vi "Inv_Mpemba1_QPDcali.vi"() -> ()   [LabVIEW 2019]
uses:
  <vilib>/eio/EIONode/EIONode.xnode
  <vilib>/rvi/eio/common/nirviEmuTemplateMethod_errors.vi
  <vilib>/eio/EIOPropertyNode/EIOPropertyNode.xnode
  <vilib>/rvi/eio/common/nirviEmuTemplatePropertyGet_errors.vi
  <vilib>/rvi/eio/common/nirviEmuTemplatePropertyGet_noerrors.vi
  <vilib>/rvi/eio/common/nirviEmuTemplatePropertySet_errors.vi
  <vilib>/rvi/eio/common/nirviEmuTemplatePropertySet_noerrors.vi
  <vilib>/rvi/DataTransferAndStorage/Container/XNode/niFpgaContainer.xnode
  <vilib>/rvi/FIFO/Fifo_Resource/nirvififoEmulationWrite.vi
  <vilib>/rvi/FIFO/Fifo_Resource/nirvififoEmulationRead.vi
  <vilib>/rvi/interface/RandomDataEmulation/nirviRandomDataFpgaReadWriteTemplate.vi
panel:
  in  "V_offset":sgl
  in  "Calibration":T1
  in  "Bias":sgl
  out "num of cycles":sgl
  in  "Xmin":sgl=-1.0
  in  "Fmax":sgl
  out "Fx out/Xcorr":sgl
  in  "Xmax":sgl=50.0
  out "Xpot":sgl format="%.2f"
  in  "Temp":i8(ring) items=["Cold", "Warm", "Hot"]
  in  "cdfnorm":sgl
  out "Saveloop":u32
  in  "Enum":enum8{"No FB", "FB"}(ring)
  in  "MobX(px/V)":sgl
  in  "1/Xcali":sgl
  in  "Feedback parameters":T2
  in  "DX":sgl
  in  "DW":cluster{"xm":sgl, "Eb":sgl, "Tau":sgl, "dE":sgl}={"xm"=0.0, "Eb"=0.0, "Tau"=50.0, "dE"=0.0}
  in  "Xmean":sgl
  in  "Calibration ON/OFF":bool
  in  "Frequency":u32=100000
  in  "wait time":sgl=35.0
  in  "Triangle wave":T3={"signal offset_X"=5.0, "Scale X"=0.0, "signal offset_Y"=5.0, "Scale Y"=0.0, "Phase Shift"=30}
  in  "Xoffset":sgl
  in  "Yoffset":sgl
  in  "sum_offset":sgl
  in  "Normalize signal":bool=TRUE
  in  "FB Time":u8=5 caption="Feedback loop time"
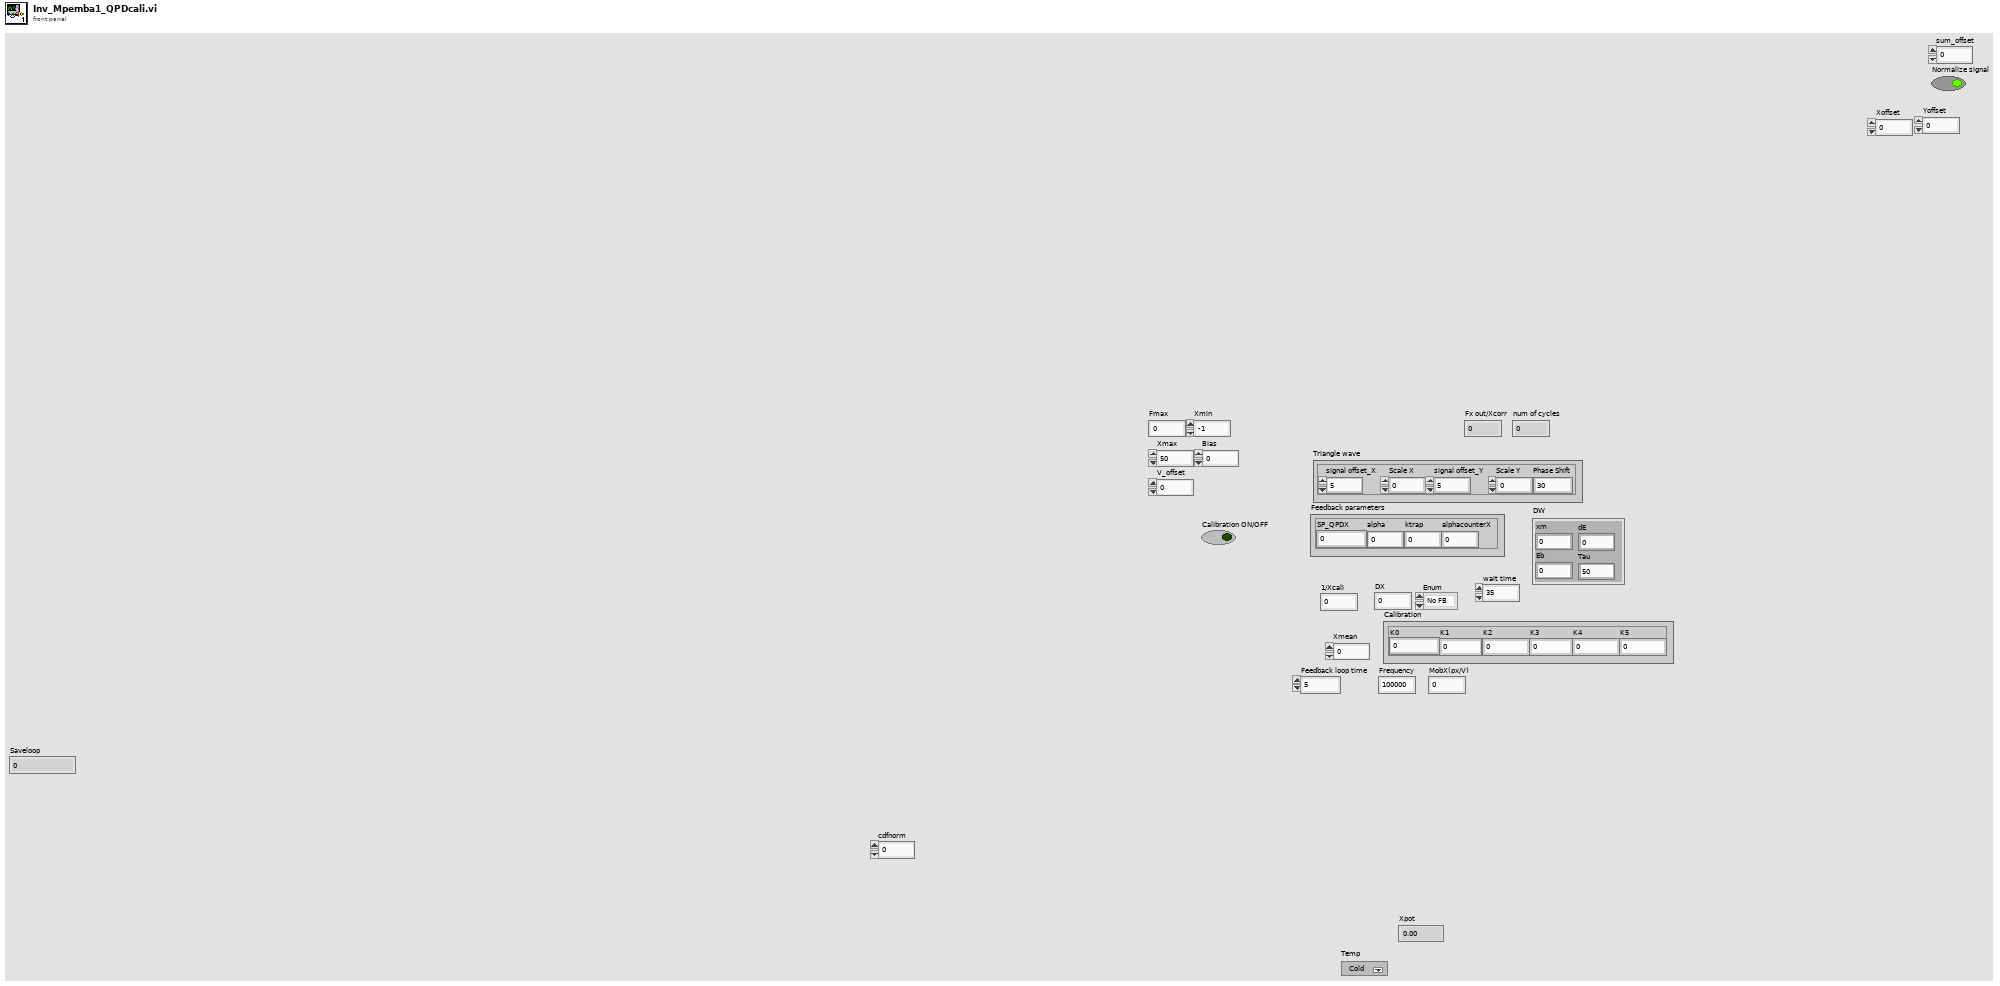
[diagram p1: front panel]
types:
  T1 = cluster{"K0":sgl, "K1":sgl, "K2":sgl, "K3":sgl, "K4":sgl, "K5":sgl}
  T2 = cluster{"SP_QPDX":sgl, "alpha":sgl, "ktrap":sgl, "alphacounterX":sgl}
  T3 = cluster{"signal offset_X":sgl, "Scale X":sgl, "signal offset_Y":sgl, "Scale Y":sgl, "Phase Shift":u32}
  T4 = enum8{"+/- 10 V", "+/- 5 V", "+/- 2 V", "+/- 1 V"}
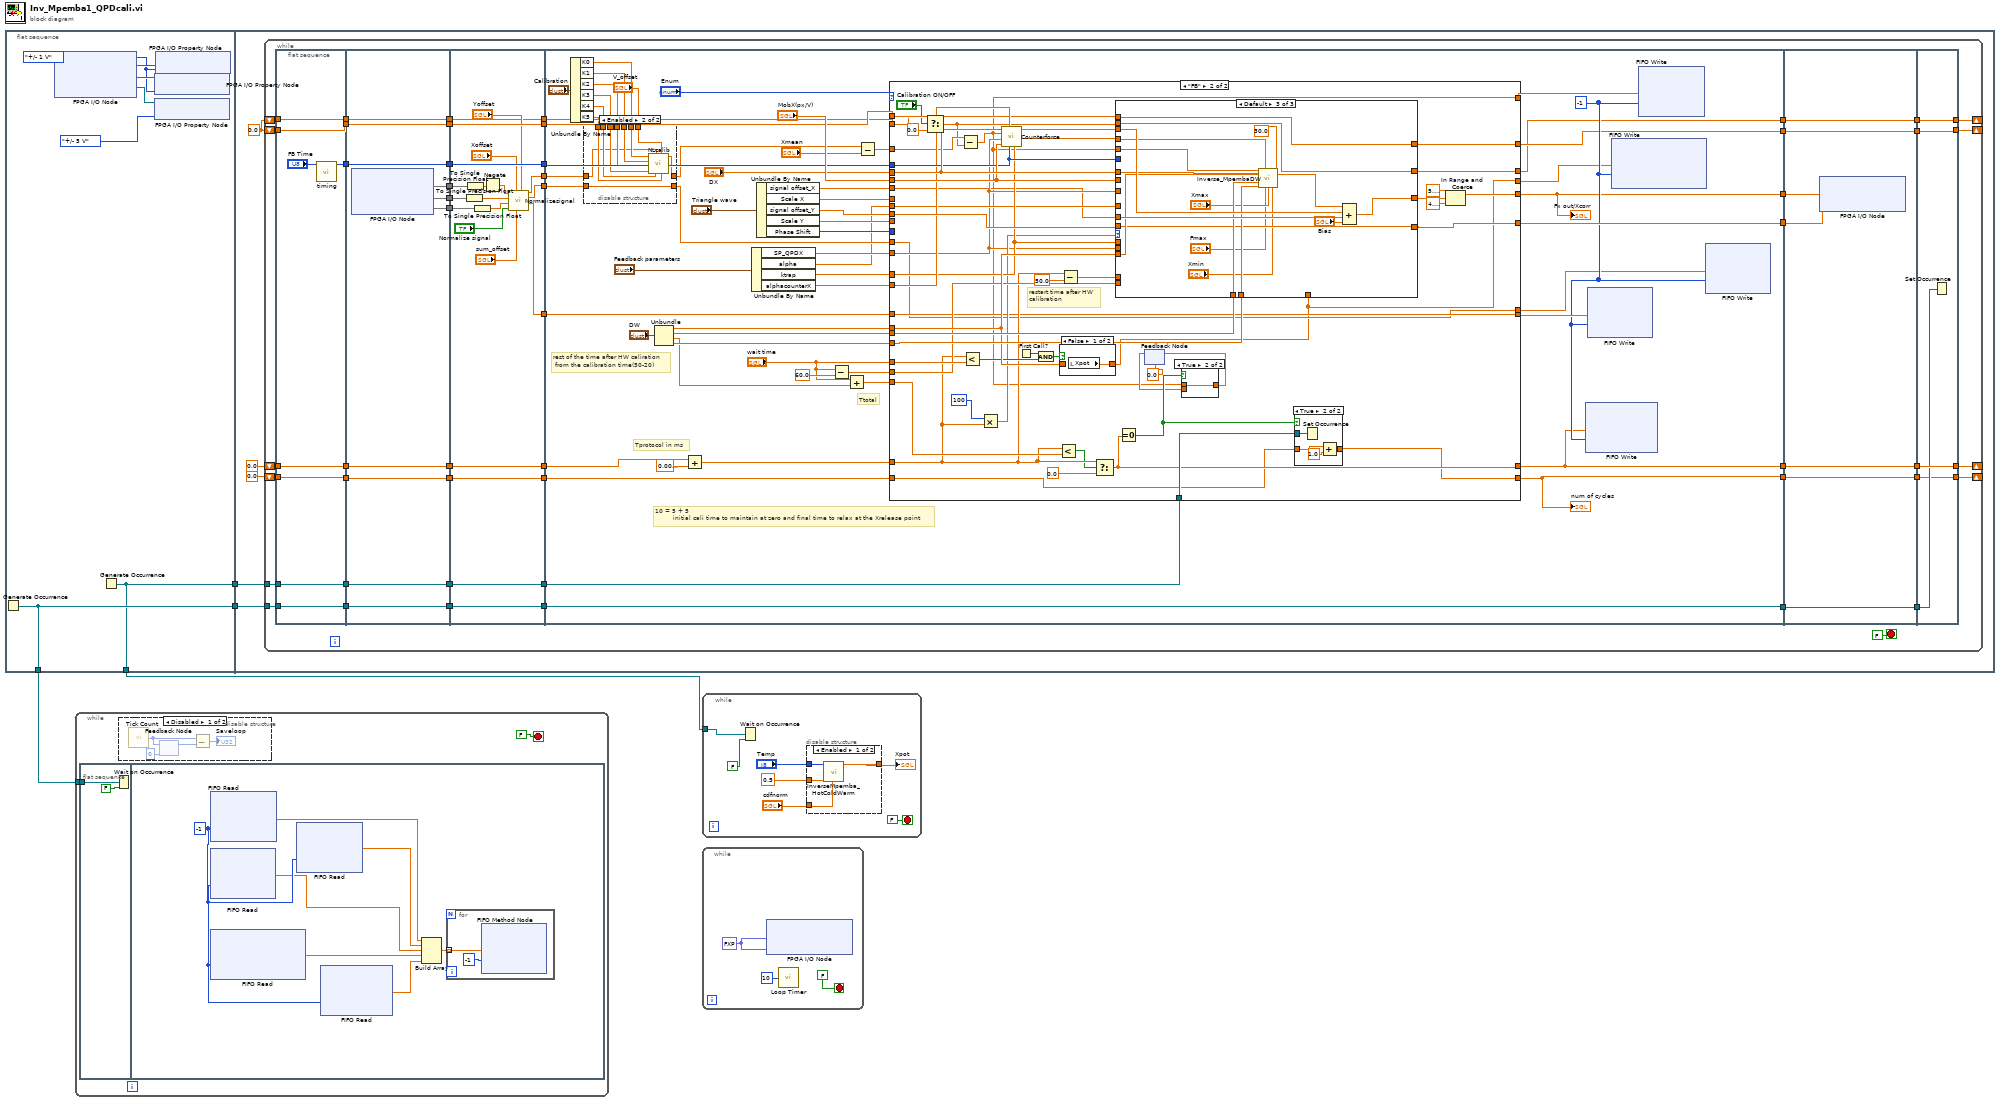
[diagram p0: block diagram]
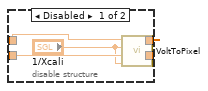
[diagram p2: hidden frame]
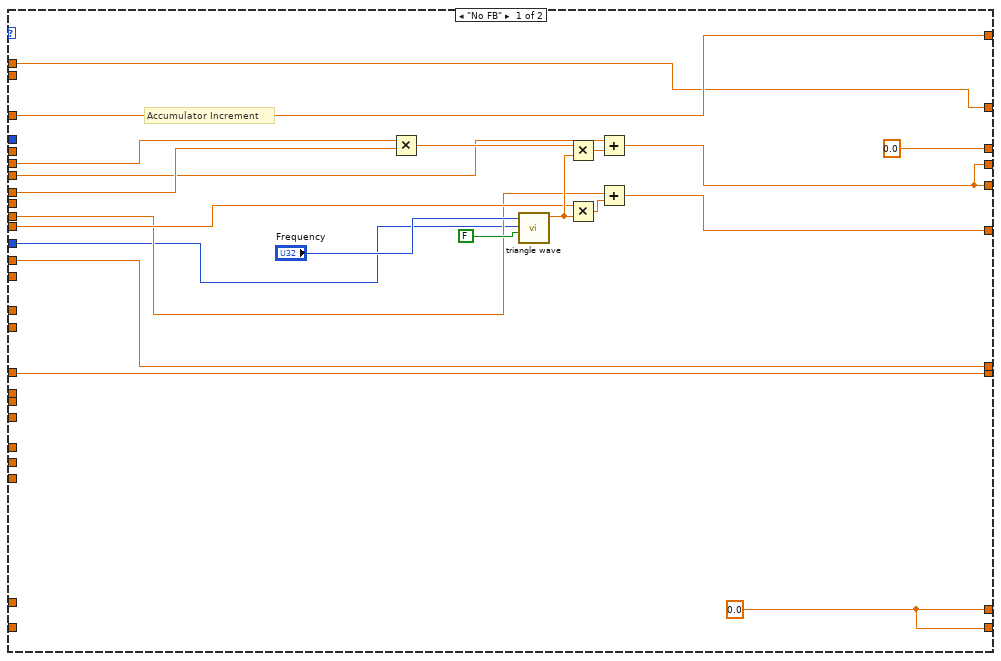
[diagram p3: hidden frame]
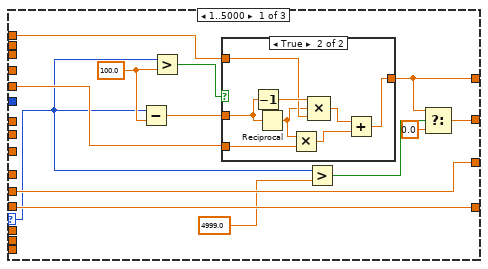
[diagram p4: hidden frame]
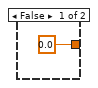
[diagram p5: hidden frame]
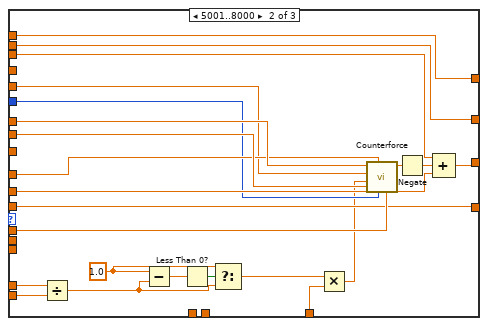
[diagram p6: hidden frame]
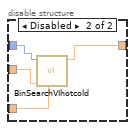
[diagram p11: hidden frame]
diagram:
  n1 = flat-sequence {
    tunnel: [w6] -> w2
    tunnel: [w5] -> w1
    tunnel: [w6] -> w4
    tunnel: [w5] -> w3
    tunnel: w2 -> [w16]
    tunnel: w1 -> [w15]
    frame #0 {
      w8 = T4."+/- 1 V" ("Voltage Range")
      n2 = Generate Occurrence() -> (w6:refnum<k4>)
      n3 = xnode "FPGA I/O Node"() -> ("FPGA I/O Out"=w11:refnum<k21>, "FPGA I/O Out"=w9:refnum<k21>, "FPGA I/O Out"=w10:refnum<k21>)  [unwired: 3 in, 3 out]
      n4 = Generate Occurrence() -> (w5:refnum<k4>)
      n5 = xnode "FPGA I/O Property Node"("FPGA I/O In"=w9, "Voltage Range"=w8) -> ()  [unwired: 1 out]
      n6 = xnode "FPGA I/O Property Node"("FPGA I/O In"=w10, "Voltage Range"=T4."+/- 5 V") -> ()  [unwired: 1 out]
      n7 = xnode "FPGA I/O Property Node"("FPGA I/O In"=w11, "Voltage Range"=w8) -> ()  [unwired: 1 out]
    }
    frame #1 {
      w12 = sgl 0.0
      n8 = while {
        tunnel: w16 -> [w47]
        shift-right: [w52] -> _
        shift-left: sgl 0.0 -> [w51]
        tunnel: w15 -> [w38]
        shift-right: [w35] -> _
        shift-left: w12 -> [w33]
        shift-right: [w28] -> _
        shift-left: sgl 0.0 ("f") -> [w26]
        shift-right: [w21] -> _
        shift-left: w12 -> [w20]
        stop <- FALSE ("stop") stop-if-true
        n9 = flat-sequence {
          tunnel: [w73] -> w55
          tunnel: w51 -> [w72]
          tunnel: [w72] -> w50
          tunnel: w47 -> [w71]
          tunnel: [w71] -> w46
          tunnel: [w70] -> w39
          tunnel: w38 -> [w70]
          tunnel: [w69] -> w34
          tunnel: w33 -> [w69]
          tunnel: [w68] -> w27
          tunnel: w26 -> [w68]
          tunnel: w20 -> [w67]
          tunnel: [w67] -> w19
          tunnel: [w84] -> w65
          tunnel: [w83] -> w63
          tunnel: [w82] -> w61
          tunnel: [w81] -> w56
          tunnel: w55 -> [w81]
          tunnel: w50 -> [w80]
          tunnel: [w80] -> w49
          tunnel: w46 -> [w79]
          tunnel: [w79] -> w45
          tunnel: [w78] -> w40
          tunnel: w39 -> [w78]
          tunnel: w34 -> [w77]
          tunnel: [w77] -> w31
          tunnel: w27 -> [w76]
          tunnel: [w76] -> w25
          tunnel: w19 -> [w75]
          tunnel: [w75] -> w18
          tunnel: w65 -> [w92]
          tunnel: [w104] -> w64
          tunnel: w63 -> [w91]
          tunnel: [w103] -> w62
          tunnel: w61 -> [w89]
          tunnel: [w102] -> w60
          tunnel: [w105] -> w57
          tunnel: w56 -> [w105]
          tunnel: w49 -> [w101]
          tunnel: [w101] -> w48
          tunnel: w45 -> [w100]
          tunnel: [w100] -> w44
          tunnel: [w99] -> w41
          tunnel: w40 -> [w99]
          tunnel: [w97] -> w32
          tunnel: w31 -> [w97]
          tunnel: w25 -> [w96]
          tunnel: [w96] -> w24
          tunnel: w18 -> [w87]
          tunnel: [w87] -> w17
          tunnel: w64 -> [w159]
          tunnel: w62 -> [w158]
          tunnel: w60 -> [w153]
          tunnel: [w114] -> w59
          tunnel: [w163] -> w58
          tunnel: w57 -> [w160]
          tunnel: [w133] -> w54
          tunnel: w48 -> [w155]
          tunnel: w44 -> [w146]
          tunnel: [w146] -> w42
          tunnel: w41 -> [w140]
          tunnel: [w135] -> w37
          tunnel: w32 -> [w134]
          tunnel: [w116] -> w30
          tunnel: w24 -> [w132]
          tunnel: [w118] -> w23
          tunnel: w17 -> [w117]
          tunnel: w58 -> [w328]
          tunnel: w59 -> [w329]
          tunnel: w54 -> [w327]
          tunnel: [w327] -> w53
          tunnel: [w326] -> w43
          tunnel: w42 -> [w326]
          tunnel: w37 -> [w325]
          tunnel: [w325] -> w36
          tunnel: w30 -> [w324]
          tunnel: [w324] -> w29
          tunnel: w23 -> [w323]
          tunnel: [w323] -> w22
          tunnel: w53 -> [w334]
          tunnel: [w334] -> w52
          tunnel: w43 -> [w333]
          tunnel: [w332] -> w35
          tunnel: w36 -> [w332]
          tunnel: w29 -> [w331]
          tunnel: [w331] -> w28
          tunnel: w22 -> [w330]
          tunnel: [w330] -> w21
          frame #0 {
            n10 = call "timing.vi"("Feedback loop time"="FB Time") -> ("Feedback Loop time"=w73:u32)  [unwired: 10 in]
          }
          frame #1 {
            n11 = xnode "FPGA I/O Node"() -> ("Connector1/AI2"=w84, "Connector1/AI4"=w83, "Connector1/AI5"=w82)  [unwired: 3 in, 3 out]
          }
          frame #2 {
            n12 = To Single Precision Float(number=w91) -> (single precision float=w90:sgl)
            n13 = To Single Precision Float(number=w92) -> (single precision float=w86:sgl)
            n14 = To Single Precision Float(number=w89) -> (single precision float=w88:sgl)
            n15 = Negate(x=w86) -> (-x=w85:sgl)
            n16 = call "Normalizesignal.vi"("Yoffset"="Yoffset", "sum_offset"="sum_offset", "Xoffset"="Xoffset", "Normalize signal"="Normalize signal", "Sum"=w88, "Y"=w90, "X"=w85) -> ("Sum"=w102:sgl, "Y"=w103:sgl, "X"=w104:sgl)  [unwired: 2 in]
          }
          frame #3 {
            w136 = -1 ("Timeout")
            # "rest of the time after HW caliration\n from the calibration time(50-20)"
            # "10 = 5 + 5\n         initial cali time to maintain at zero and final time to relax at the Xrelease point"
            # "Tprotocol in ms"
            # "Ttotal"
            n17 = Unbundle By Name("Calibration") -> ("K0"=w111:sgl, "K1"=w110:sgl, "K2"=w109:sgl, "K3"=w108:sgl, "K4"=w107:sgl, "K5"=w106:sgl)
            n18 = disable-structure shown="Enabled" {
              disable-tunnel: w159 -> [w168 w170]
              disable-tunnel: w158 -> [w167 w178]
              disable-tunnel: [w166 w178] -> w157
              disable-tunnel: [w165 w169] -> w143
              disable-tunnel: "V_offset" -> [_ w177]
              disable-tunnel: w111 -> [_ w176]
              disable-tunnel: w110 -> [_ w175]
              disable-tunnel: w109 -> [_ w174]
              disable-tunnel: w108 -> [_ w173]
              disable-tunnel: w107 -> [_ w172]
              disable-tunnel: w106 -> [_ w171]
              frame Disabled {
                n19 = call "VoltToPixel.vi"("1/(QPDY/px)"="1/Xcali", "Normalized Y"=w167, "1/(QPDX/px)"="1/Xcali", "Normalized X"=w168) -> ("Ypx"=w166:sgl, "Xpx"=w165:sgl)  [unwired: 6 in]
              }
              frame Enabled {
                n20 = call "NLcalib.vi"("K5"=w171, "V_offset"=w177, "K4"=w172, "Volt QPD"=w170, "K3"=w173, "K2"=w174, "K1"=w175, "K0"=w176) -> ("pixels"=w169:sgl)  [unwired: 3 in]
              }
            }
            n21 = Unbundle("DW") -> ("xm"=w141:sgl, "Eb"=w154:sgl, "Tau"=w120:sgl, "dE"=w148:sgl)
            n22 = Add(x=w155, y=sgl 0.01) -> (x+y=w147:sgl)
            n23 = Unbundle By Name("Feedback parameters") -> ("SP_QPDX"=w124:sgl, "alpha"=w121:sgl, "ktrap"=w122:sgl, "alphacounterX"=w123:sgl)
            n24 = Unbundle By Name("Triangle wave") -> ("signal offset_X"=w128:sgl, "Scale X"=w130:sgl, "signal offset_Y"=w127:sgl, "Scale Y"=w129:sgl, "Phase Shift"=w126:u32)
            n25 = Subtract(x="wait time", y=sgl 60.0) -> (x-y=w139:sgl)
            n26 = Add(x="wait time", y=w120) -> (x+y=w156:sgl)
            n27 = Subtract(x=w143, y="Xmean") -> (x-y=w151:sgl)
            n28 = case shown="\"FB\"" "Enum" {
              tunnel: w151 -> [w196 w204]
              tunnel: [w179 w224] -> w114
              tunnel: [w190 w216] -> w163
              tunnel: [w196 w202] -> w150
              tunnel: [w198 w209] -> w149
              tunnel: w153 -> [w198 w209]
              tunnel: w157 -> [w197 w206]
              tunnel: [w197 w206] -> w119
              tunnel: "MobX(px/V)" -> [w189 w247]
              tunnel: w160 -> [_ w230]
              tunnel: "DX" -> [_ w248]
              tunnel: w141 -> [_ w243]
              tunnel: w154 -> [_ w249]
              tunnel: w147 -> [_ w218]
              tunnel: w156 -> [_ w232]
              tunnel: [w181 w241] -> w133
              tunnel: w148 -> [_ w246]
              tunnel: w140 -> [_ w242]
              tunnel: "wait time" -> [_ w238]
              tunnel: w139 -> [_ w229]
              tunnel: [w188 w200] -> w135
              tunnel: w134 -> [w188 w212]
              tunnel: [w181 w226] -> w116
              tunnel: w132 -> [_ w225]
              tunnel: w130 -> [w186 _]
              tunnel: w129 -> [w185 _]
              tunnel: w128 -> [w184 w205]
              tunnel: w127 -> [w183 w223]
              tunnel: w126 -> [w182 _]
              tunnel: w124 -> [_ w213]
              tunnel: w123 -> [_ w222]
              tunnel: w122 -> [_ w221]
              tunnel: w121 -> [_ w220]
              tunnel: [sgl 0.0 ("f") w201] -> w118
              tunnel: w117 -> [_ w207]
              tunnel: [w179 w199] -> w115
              frame "No FB" {
                w181 = sgl 0.0 ("f")
                # "Accumulator Increment"
                n29 = Multiply(x=w189, y=w186) -> (x*y=w194:sgl)
                n30 = call "triangle wave.vi"("Reset Accumulator_TW"=FALSE, "phase shift"=w182, "Frequency"="Frequency") -> ("Tri wave out"=w191:sgl)  [unwired: 8 in]
                n31 = Multiply(x=w194, y=w191) -> (x*y=w193:sgl)
                n32 = Multiply(x=w185, y=w191) -> (x*y=w195:sgl)
                n33 = Add(x=w184, y=w193) -> (x+y=w179:sgl)
                n34 = Add(x=w183, y=w195) -> (x+y=w190:sgl)
              }
              frame "FB" {
                # "restart time after HW\ncalibration"
                n35 = Select(t=w207, s="Calibration ON/OFF", f=sgl 0.0) -> (s? t:f=w203:sgl)
                n36 = Subtract(x=w204, y=w203) -> (x-y=w202:sgl)
                n37 = Less?(x=w218, y=w238) -> (x < y?=w234:bool)
                n38 = Multiply(x=i16 100, y=w218) -> (x*y=w217:sgl)
                n39 = call "Counterforce.vi"("ktrap"=w221, "Ts"=w230, "alphacounterX"=w222, "mobX(px/V)"=w247, "SP_X"=w213, "Xpx"=w202, "Dx"=w248) -> ("ktrap*mob"=w239:sgl, "counter Force"=w240:sgl)  [unwired: 2 in, 1 out]
                n40 = First Call?() -> (First Call?: T/F=w245:bool)
                n41 = And(x=w245, y=w234) -> (x .and. y?=w244:bool)
                n42 = Less?(x=w218, y=w232) -> (x < y?=w208:bool)
                n43 = case shown="False" w244 {
                  tunnel: [w321 w322] -> w199
                  tunnel: w243 -> [_ w322]
                  frame False {
                    n44 = local read "Xpot"() -> (w321:sgl)
                  }
                  frame True {
                  }
                }
                n45 = Subtract(x=w218, y=sgl 50.0) -> (x-y=w227:sgl)
                n46 = Select(t=w218, s=w208, f=sgl 0.0) -> (s? t:f=w241:sgl)
                n47 = case shown="Default" w217 {
                  selector: w217 -> [w256 _ _]
                  tunnel: w202 -> [w258 w275 w305]
                  tunnel: w248 -> [_ w295 w300]
                  tunnel: w247 -> [_ w294 _]
                  tunnel: [w257 w293 w308] -> w219
                  tunnel: [w262 w289 w307] -> w216
                  tunnel: w221 -> [_ w290 _]
                  tunnel: w223 -> [w262 w289 w307]
                  tunnel: w205 -> [w257 w286 w313]
                  tunnel: w220 -> [_ w288 _]
                  tunnel: w243 -> [_ _ w311]
                  tunnel: w249 -> [_ _ w310]
                  tunnel: w240 -> [_ w287 w312]
                  tunnel: w239 -> [_ _ w302]
                  tunnel: w246 -> [_ _ w309]
                  tunnel: w213 -> [_ _ _]
                  tunnel: [w253 w276 w306] -> w200
                  tunnel: w212 -> [w259 w276 w306]
                  tunnel: w230 -> [_ w285 _]
                  tunnel: w199 -> [_ w284 _]
                  tunnel: w227 -> [_ w278 _]
                  tunnel: w229 -> [_ w277 _]
                  tunnel: w213 -> [_ _ _]
                  tunnel: [w251 w274 w303] -> w201
                  tunnel: w203 -> [_ w274 w303]
                  frame 1..5000 {
                    w263 = sgl 100.0 ("y")
                    n48 = Subtract(x=w256, y=w263) -> (x-y=w260:sgl)
                    n49 = Greater?(x=w256, y=w263) -> (0:w261:bool)
                    n50 = case shown="True" w261 {
                      tunnel: [sgl 0.0 w266] -> w253
                      tunnel: w260 -> [_ w272]
                      tunnel: w259 -> [_ w270]
                      tunnel: w258 -> [_ w269]
                      frame False {
                      }
                      frame True {
                        n51 = Decrement(x=w272) -> (x-1=w271:sgl)
                        n52 = Reciprocal(x=w272) -> (1/x=w265:sgl)
                        n53 = Multiply(x=w265, y=w269) -> (x*y=w267:sgl)
                        n54 = Compound Arithmetic op=MULTIPLY(w271, w265, w270) -> (w268:sgl)
                        n55 = Add(x=w268, y=w267) -> (x+y=w266:sgl)
                      }
                    }
                    n56 = Greater?(x=w256, y=sgl 4999.0) -> (0:w254:bool)
                    n57 = Select(t=w253, s=w254, f=sgl 0.0) -> (s? t:f=w251:sgl)
                  }
                  frame 5001..8000 {
                    w280 = sgl 1.0 ("y")
                    n58 = Divide(x=w278, y=w277) -> (x/y=w279:sgl)
                    n59 = Subtract(x=w280, y=w279) -> (x-y=w281:sgl)
                    n60 = Less Than 0?(x=w281) -> (x < 0?=w282:bool)
                    n61 = Select(t=w280, s=w282, f=w279) -> (s? t:f=w283:sgl)
                    n62 = Multiply(x=w283, y=w284) -> (x*y=w273:sgl)
                    n63 = call "Counterforce.vi"("ktrap"=w290, "Ts"=w285, "alphacounterX"=w288, "mobX(px/V)"=w294, "SP_X"=w273, "Xpx"=w275, "Dx"=w295) -> ("counter Force"=w292:sgl)  [unwired: 2 in, 2 out]
                    n64 = Negate(x=w292) -> (-x=w291:sgl)
                    n65 = Compound Arithmetic op=ADD(w287, w291, w286) -> (w293:sgl)
                  }
                  frame Default {
                    n66 = call "Inverse_MpembaDW.vi"("Xpos"=w305, "ktrap*mob"=w302, 2:w300, 4:sgl 30.0 ("Force"), "Xm"=w311, "Eb"=w310, "dE"=w309, "Fmax"="Fmax", "Xmax"="Xmax", "Xmin"="Xmin") -> ("DWvolt"=w304:sgl)  [unwired: 5 in]
                    n67 = Compound Arithmetic op=ADD(w304, w312, w313, "Bias") -> (w308:sgl)
                  }
                }
                n68 = Equal To 0?(x=w241) -> (x = 0?=w237:bool)
                n69 = feedback #1(sgl 0.0) -> (w235:sgl)
                n70 = case shown="True" w237 {
                  tunnel: w202 -> [_ w320]
                  tunnel: [w319 w320] -> w236
                  tunnel: w235 -> [w319 _]
                  frame False {
                  }
                  frame True {
                  }
                }
                n71 = feedback-in #1(w236) -> ()
                n72 = case shown="True" w237 {
                  tunnel: w242 -> [_ w318]
                  tunnel: [w314 w317] -> w226
                  tunnel: w225 -> [w314 w316]
                  frame False {
                  }
                  frame True {
                    n73 = Set Occurrence(w318) -> ()
                    n74 = Add(x=w316, y=sgl 1.0) -> (x+y=w317:sgl)
                  }
                }
                n75 = In Range and Coerce(upper limit=sgl 5.1, x=w219, lower limit=sgl 4.9) -> (coerced(x)=w224:sgl)  [unwired: 1 out]
              }
            }
            "Fx out/Xcorr" <- w114
            "num of cycles" <- w116
            n76 = xnode ("FIFO Write")("Element"=w133, "Timeout"=w136) -> ()  [unwired: 1 in, 2 out]
            n77 = xnode ("FIFO Write")("Element"=w149, "Timeout"=w136) -> ()  [unwired: 1 in, 2 out]
            n78 = xnode ("FIFO Write")("Element"=w115, "Timeout"=w136) -> ()  [unwired: 1 in, 2 out]
            n79 = xnode ("FIFO Write")("Element"=w150, "Timeout"=w136) -> ()  [unwired: 1 in, 2 out]
            n80 = xnode ("FIFO Write")("Element"=w119, "Timeout"=w136) -> ()  [unwired: 1 in, 2 out]
          }
          frame #4 {
            n81 = xnode "FPGA I/O Node"("Connector1/AO7"=w329, "Connector1/AO6"=w328) -> ()  [unwired: 2 in, 2 out]
          }
          frame #5 {
            n82 = Set Occurrence(w333) -> ()
          }
        }
      }
    }
  }
  n83 = while {
    tunnel: w4 -> [w335]
    stop <- FALSE stop-if-true
    n84 = flat-sequence {
      tunnel: w335 -> [w342]
      frame #0 {
        n85 = Wait on Occurrence(1:FALSE ("ignore previous (T)"), 2:w342) -> ()  [unwired: 1 in, 1 out]
      }
      frame #1 {
        w345 = -1 ("Timeout")
        n86 = xnode ("FIFO Read")("Timeout"=w345) -> ("Element"=w343:sgl)  [unwired: 1 in, 2 out]
        n87 = xnode ("FIFO Read")("Timeout"=w345) -> ("Element"=w346:sgl)  [unwired: 1 in, 2 out]
        n88 = xnode ("FIFO Read")("Timeout"=w345) -> ("Element"=w347:sgl)  [unwired: 1 in, 2 out]
        n89 = xnode ("FIFO Read")("Timeout"=w345) -> ("Element"=w344:sgl)  [unwired: 1 in, 2 out]
        n90 = xnode ("FIFO Read")("Timeout"=w345) -> ("Element"=w348:sgl)  [unwired: 1 in, 2 out]
        n91 = Build Array(w347, w344, w343, w346, w348) -> (w349:sgl[])
        n92 = for {
          tunnel: w349 -> [w351] mode=indexing
          n93 = xnode ("FIFO Method Node")("Element"=w351, "Timeout"=-1) -> ()  [unwired: 1 in, 2 out]
        }
      }
    }
    n94 = disable-structure shown="Disabled" {
      frame Disabled {
        n95 = call "Tick Count"() -> ("Tick Count(uSec)"=w340:u32)
        n96 = feedback #2(u32 0 ("Tick Count(uSec)")) -> (w339:u32)
        n97 = feedback-in #2(w340) -> ()
        n98 = Subtract(x=w340, y=w339) -> (x-y=→"Saveloop":u32)
      }
      frame Enabled {
      }
    }
  }
  n99 = while {
    stop <- FALSE stop-if-true
    w352 = fxp<+,8,3> 2.5 ("Connector1/AO2")
    n100 = xnode "FPGA I/O Node"("Connector1/AO0"=w352, "Connector1/AO4"=w352) -> ()  [unwired: 2 in, 2 out]
    n101 = call "Loop Timer"("Count(uSec)"=u8 10) -> ()  [unwired: 1 out]
  }
  n102 = while {
    tunnel: w3 -> [w360]
    stop <- FALSE ("stop") stop-if-true
    n103 = Wait on Occurrence(1:FALSE ("ignore previous (T)"), 2:w360) -> ()  [unwired: 1 in, 1 out]
    n104 = disable-structure shown="Enabled" {
      disable-tunnel: [w365 w366] -> w358
      disable-tunnel: sgl 0.5 ("X0") -> [w364 w368]
      disable-tunnel: "Temp" -> [w363 w369]
      disable-tunnel: "cdfnorm" -> [w362 w367]
      frame Enabled {
        n105 = call "InverseMpemba_HotColdWarm.vi"("RN"=w362, "X0"=w364, "Ring"=w363) -> ("Xpot"=w365:sgl)  [unwired: 8 in]
      }
      frame Disabled {
        n106 = call "BinSearchVIhotcold.vi"("RN"=w367, "X0"=w368, "Ring"=w369) -> ("Xpot"=w366:sgl)  [unwired: 8 in]
      }
    }
    "Xpot" <- w358
  }
